vi "Interfaz Control.vi"() -> ()   [LabVIEW 2022 SP3]
uses:
  MQTT/mqtt_lv2013/mqtt Folder/src/class/mqtt/mqttTypedef/mqttSubscribeCluster.ctl
  MQTT/mqtt_lv2013/mqtt Folder/src/class/mqtt/mqttTypedef/mqttQOSlevel.ctl
  MQTT/mqtt_lv2013/mqtt Folder/src/class/mqtt/mqttTypedef/mqttConnectionStatus.ctl
  MQTT/mqtt_lv2013/mqtt Folder/src/class/mqtt/mqttTypedef/mqttConnectionMeta.ctl
  MQTT/mqtt_lv2013/mqtt Folder/src/class/mqtt/mqttTXqueue/mqttTXdataQueueFunction.ctl
  MQTT/mqtt_lv2013/mqtt Folder/src/class/mqtt/mqttConfigFunction.ctl
  MQTT/mqtt_lv2013/mqtt Folder/src/class/mqtt/mqttTXqueue/mqttRXsubscriptionEventFunction.ctl
  MQTT/mqtt_lv2013/mqtt Folder/src/class/mqtt/mqttTypedef/mqttBroker.ctl
  MQTT/mqtt_lv2013/mqtt Folder/src/class/mqtt/mqttTypedef/mqttConnectionFlags.ctl
  MQTT/mqtt_lv2013/mqtt Folder/src/class/mqtt/mqttTypedef/mqttWillInformation.ctl
  MQTT/mqtt_lv2013/mqtt Folder/src/class/mqtt/mqtt.lvclass
panel:
  out "Retirando pieza del escaner":bool
  in  "Numeric 2":u64
  out "Escaner Finalizo":bool
  out "publishMessageID 6":u16 format="%02x"
  in  "connMeta 6":T1
  in  "Home Brazo":bool
  out "String":string
  in  "Ir a":bool
  out "publishMessageID 5":u16 format="%02x"
  in  "connMeta 5":T1
  in  "Horizontal Pointer Slide":u32(slide)
  out "Escaner en proceso":bool
  out "publishMessageID 4":u16 format="%02x"
  in  "connMeta 4":T1
  in  "Selección Pieza a cortar":u16(ring) items=["Ninguna", "1", "2", "3", "4", "5", "6", "7", "8", "9", "10"]
  in  "Selección Pieza a imprimir":u16(ring) items=["Ninguna", "1", "2", "3", "4", "5"]
  in  "Cantidad de piezas a cortar":u16(ring) items=["Ninguna", "1", "2", "3", "4"]
  in  "Cantidad de piezas a imprimir":u16(ring) items=["Ninguna", "1", "2", "3", "4"]
  out "publishMessageID 3":u16 format="%02x"
  in  "connMeta 3":T1
  in  "Pieza a Cortar":u16(ring)
  in  "Pieza a Imprimir":u16(ring)
  in  "quit":bool
  out "Verificar Conexión":bool=TRUE
  in  "pingRequest":bool
  out "messageID":u16
  out "RX Value":string
  out "RX Topic":string
  in  "subscribe":bool
  in  "connect":bool
  out "Colocando pieza en escaner":bool
  out "Retirando pieza del Escaner 3D":bool
  out "Retirando pieza de cortadora Laser":bool
  out "Retirando pieza de Impresora 3D":bool
  out "Brazo en reposo":bool
  out "Br. Soldador en proceso":bool
  out "Pieza Posicionada":bool
  out "Cortadora en proceso":bool
  in  "Detener Impresora 5":bool
  in  "Iniciar Cortadora 6":bool
  in  "Iniciar Cortadora 5":bool
  in  "Iniciar Cortadora 4":bool
  in  "Detener Impresora 4":bool
  in  "Iniciar Escaner":bool
  in  "Detener Impresora 2":bool
  in  "Iniciar Cortadora":bool
  in  "Detener Impresora":bool
  in  "Iniciar Impresora":bool
  out "Impresora Terminó":bool
  out "publishMessageID 2":u16 format="%02x"
  in  "connMeta 2":T1
  out "Activación Proceso":bool
  out "y":string="Test"
  out "Numeric":i32
  in  "disconnect":bool
  out "sessionPresent":bool
  out "connStatus":T3
  in  "subscriptionInfo":T4[](array[typedef])=[{"Topic"="a/b", "QoS"=enum."At most once"}]
  out "subscribeMessageID":u16 format="%02x"
  out "subscribeSuccess":bool
  out "error out":errorcluster
  # "Impresora 3D"
  # "Brazo Manipulador"
  # "Cortadora Láser"
  # "Comunicación con el CIM"
  # "Escaner 3D"
  # "Brazo Soldador"
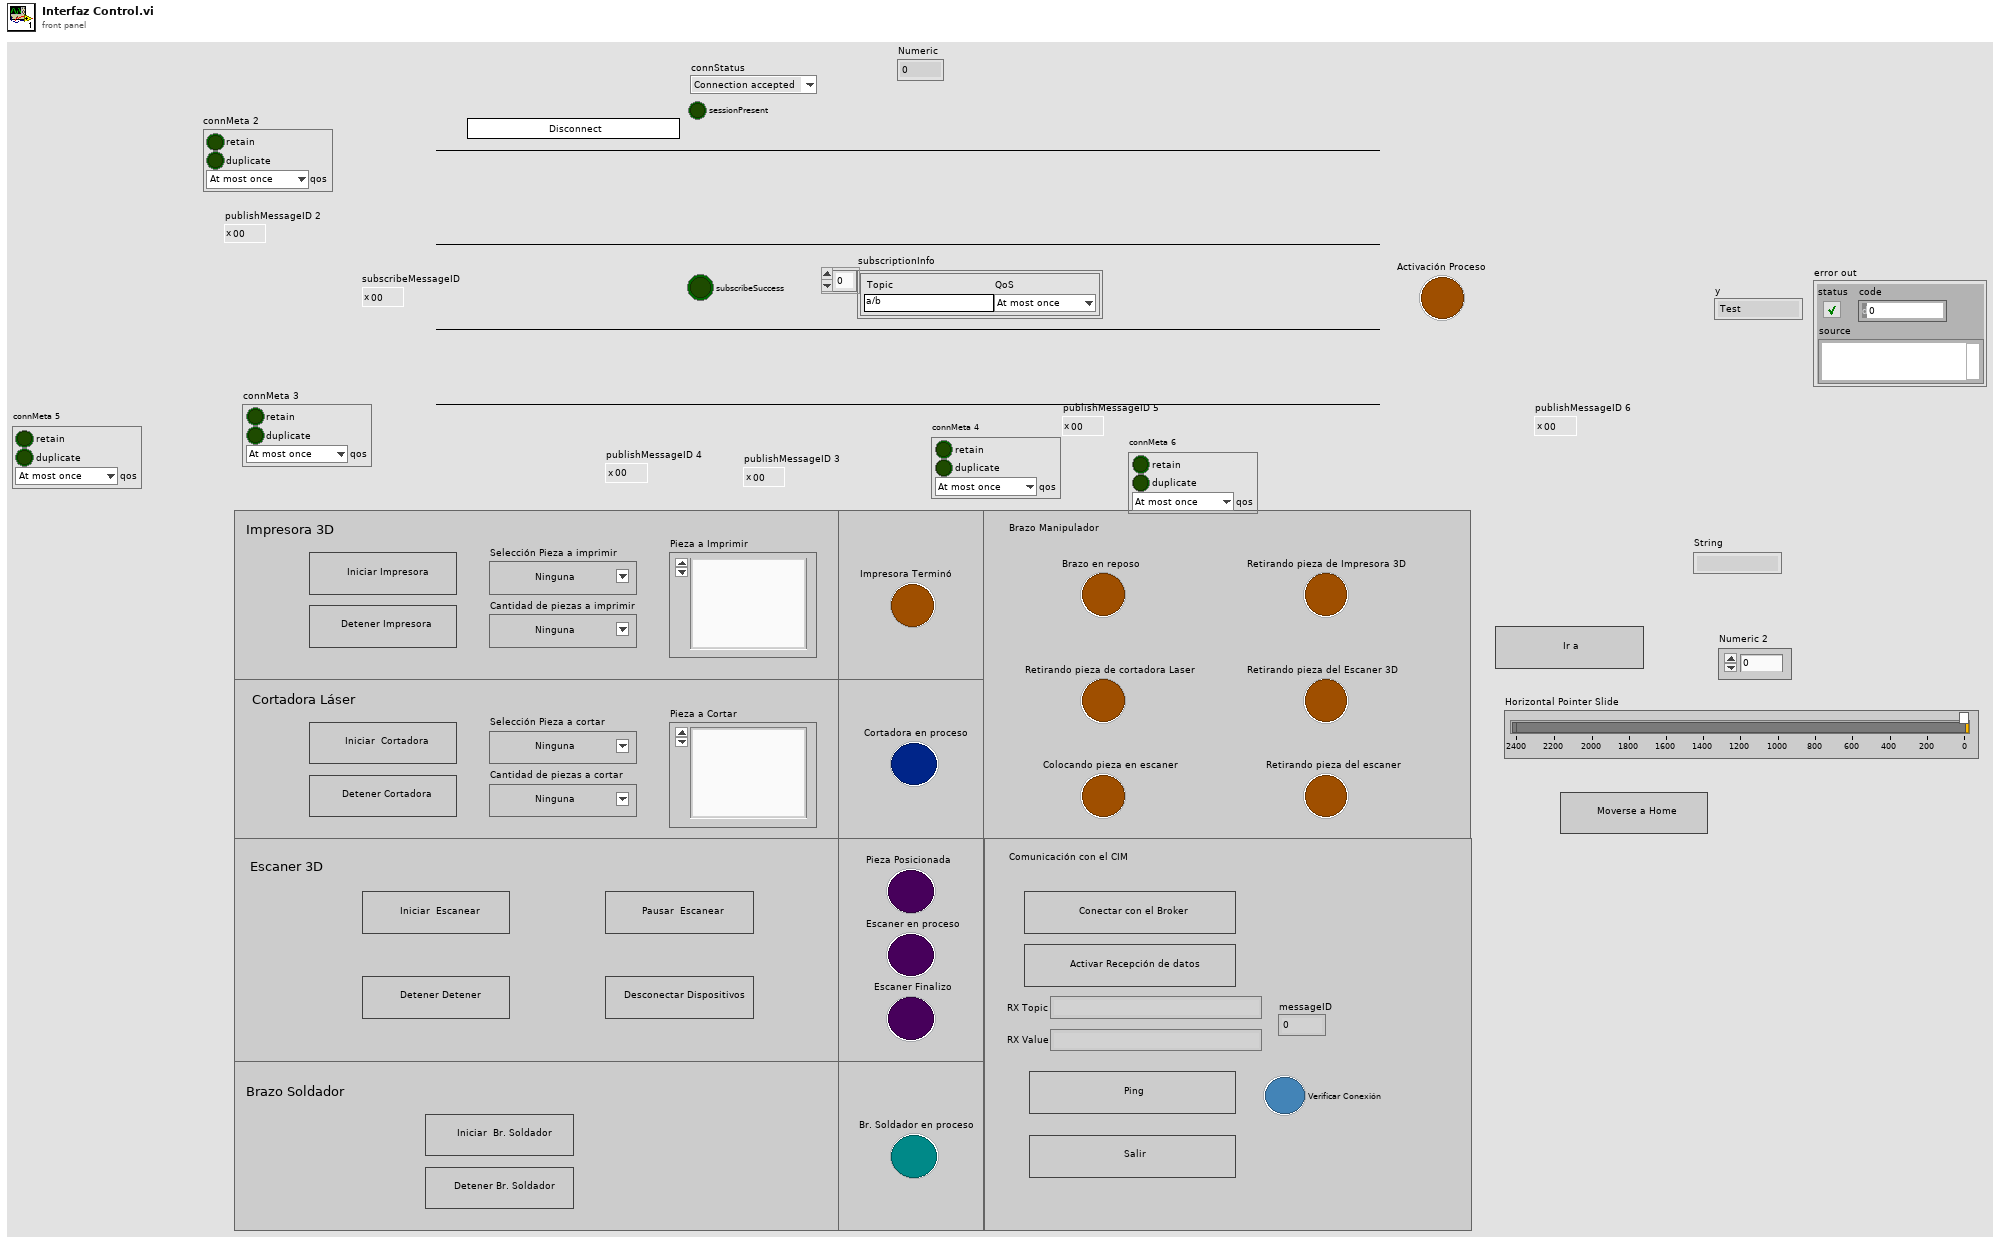
[diagram p1: front panel]
types:
  T1 = typedef "mqttConnectionMeta.ctl" = cluster{"retain":bool, "duplicate":bool, "qos":T2}
  T2 = typedef "mqttQOSlevel.ctl" = enum8{"At most once", "At least once", "Exactly once", "Reserved"}
  T3 = typedef "mqttConnectionStatus.ctl" = enum16{"Connection accepted", "Connection refused: unacceptable protocol version", "Connection refused: identifier rejected", "Connection refused: Server unavailable", "Connection refused: bad user name or password", "Connection refused: not authorized"}
  T4 = typedef "mqttSubscribeCluster.ctl" = cluster{"Topic":string, "QoS":T2}
  T5 = typedef "mqttWillInformation.ctl" = cluster{"User Name":string, "Password":string}
  T6 = typedef "mqttConnectionFlags.ctl" = cluster{"reserved":bool, "clean session":bool, "will flag":bool, "willQOS":enum8{"At most once", "At least once", "Exactly once", "Reserved"}, "will retain":bool, "password":bool, "user name":bool}
  T7 = typedef "mqttBroker.ctl" = cluster{"address":string, "port":u16, "connTimeout":i32, "writeTimeout":i32, "readTimeout":i32, "subTimeout":i32}
  T8 = typedef "mqttRXsubscriptionEventFunction.ctl" = enum16{"init", "deinit", "getEventRef", "event"}
  T9 = typedef "mqtt.lvclass/mqttConfigFunction.ctl" = enum16{"init", "deinit", "set", "get"}
  T10 = typedef "mqttTXdataQueueFunction.ctl" = enum16{"init", "deinit", "getQueue", "enqueue"}
  T11 = enum8{"Enabled", "Disabled", "Disabled and Grayed Out"}
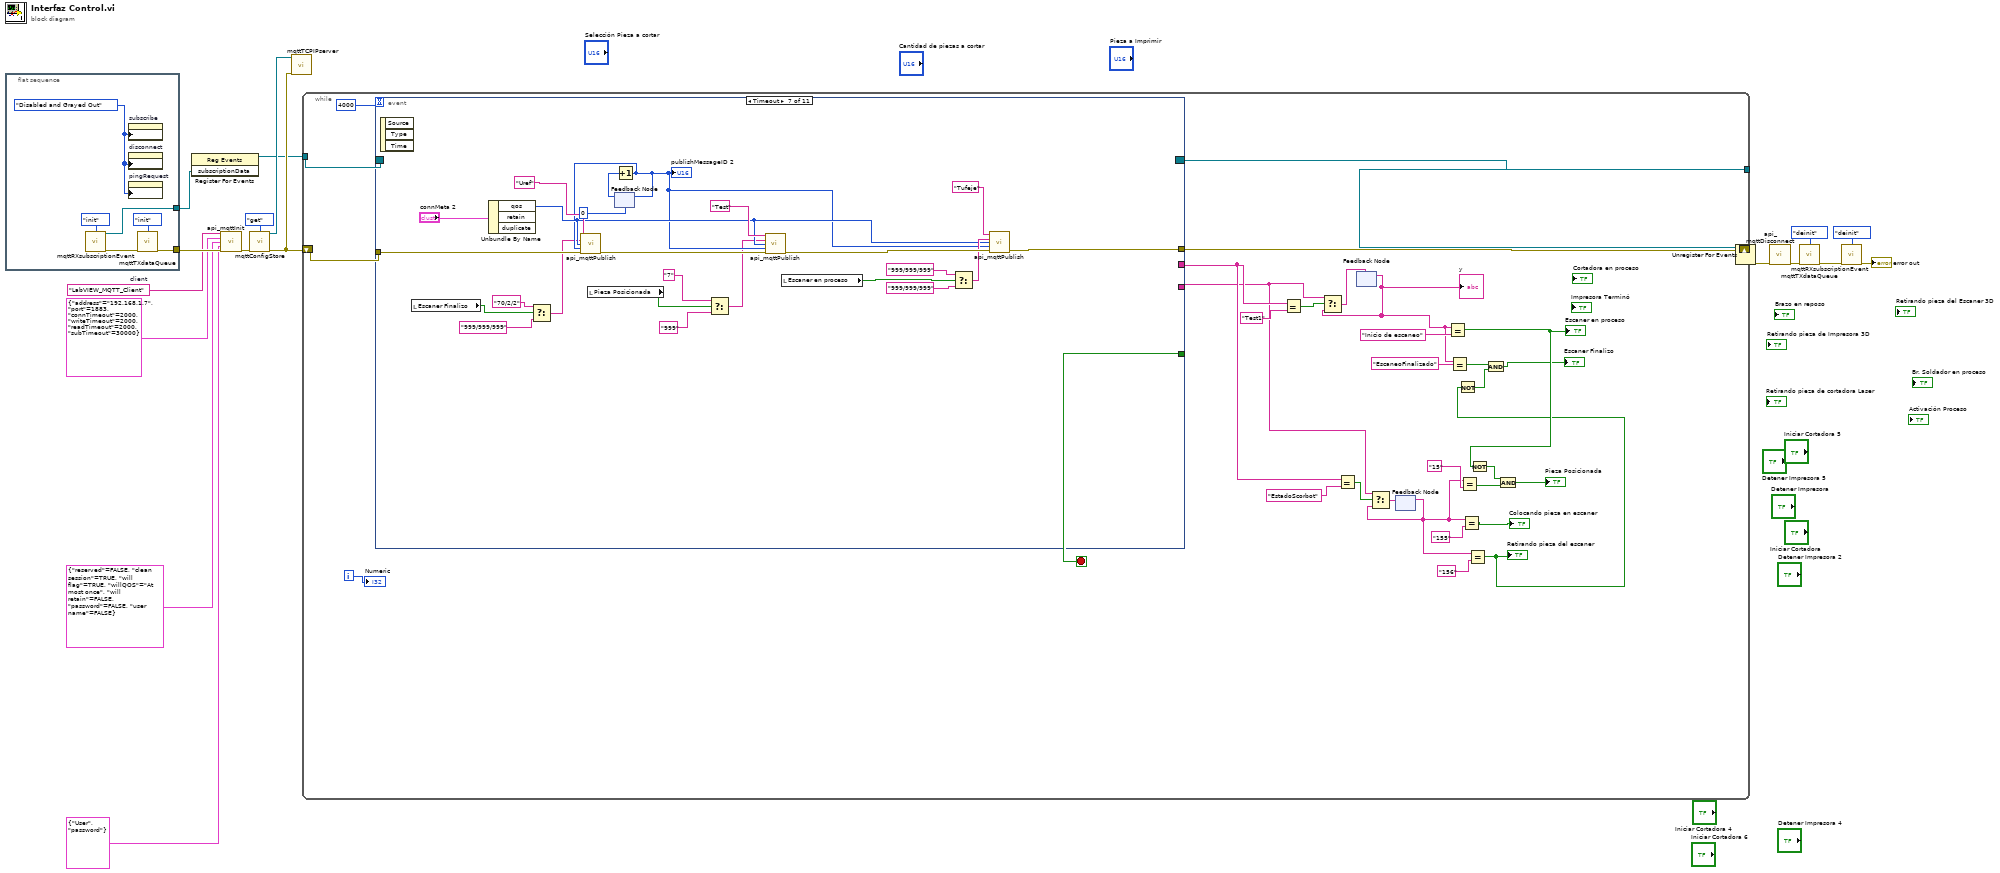
[diagram p0: block diagram]
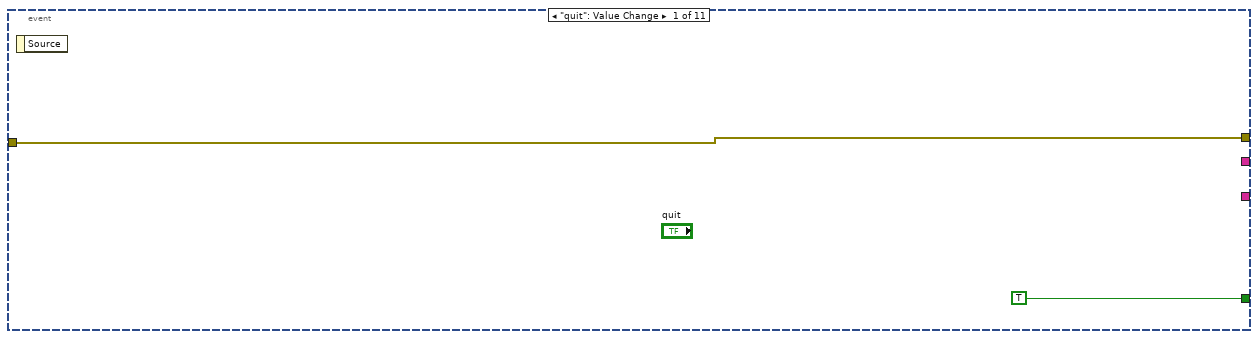
[diagram p2: hidden frame]
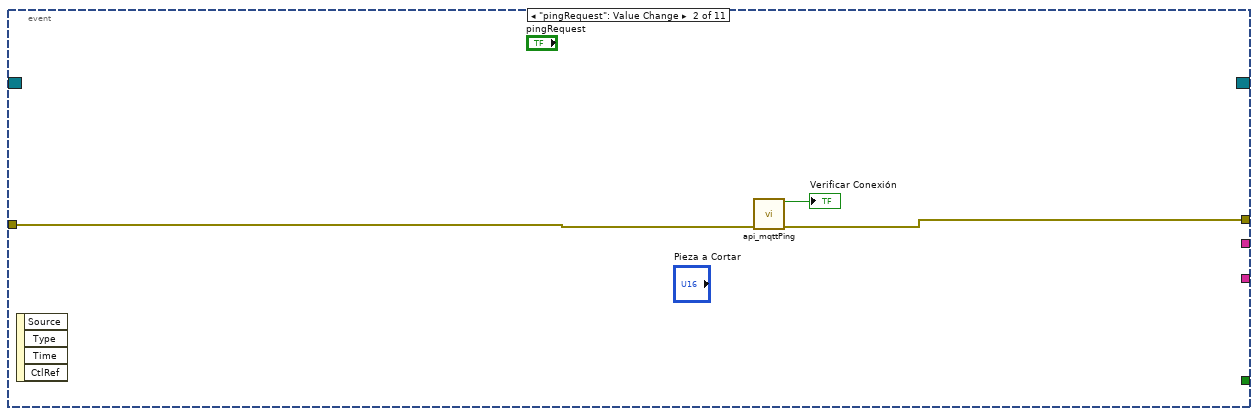
[diagram p3: hidden frame]
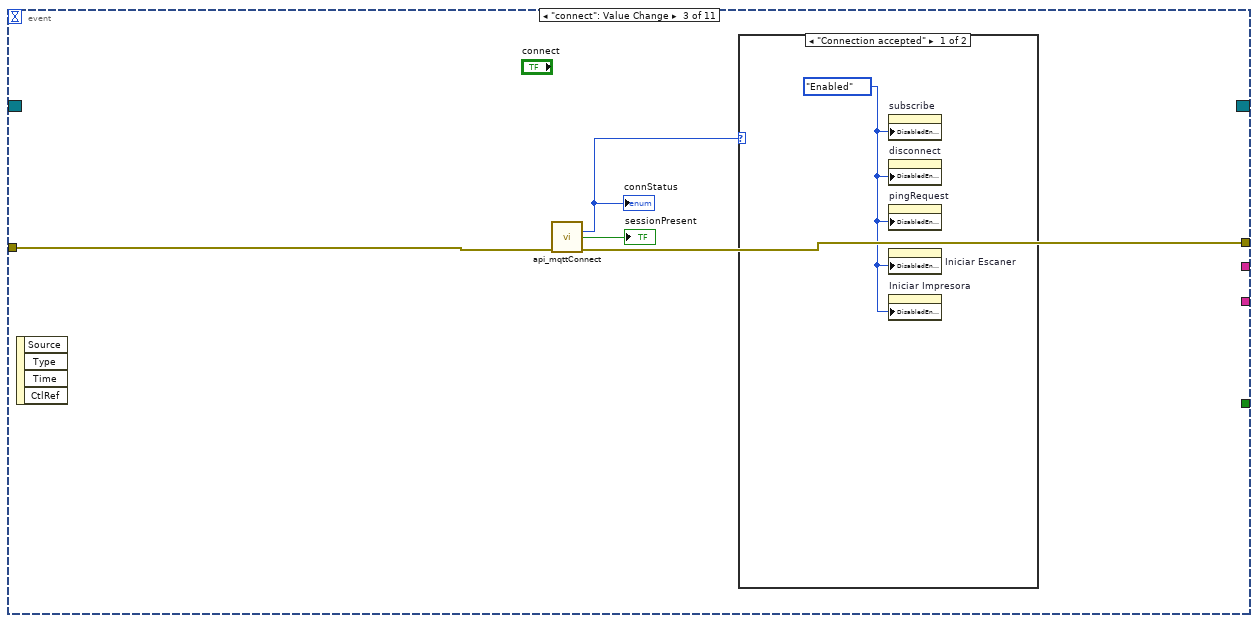
[diagram p4: hidden frame]
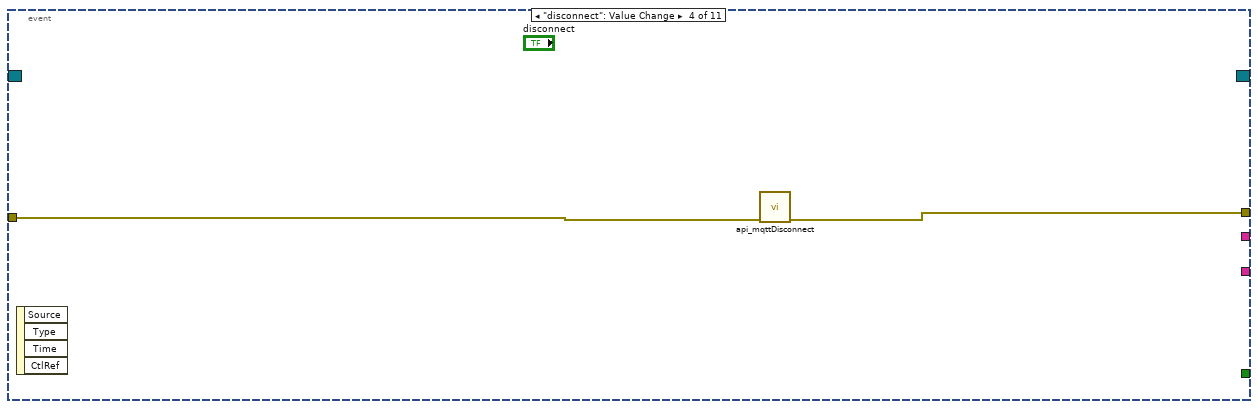
[diagram p6: hidden frame]
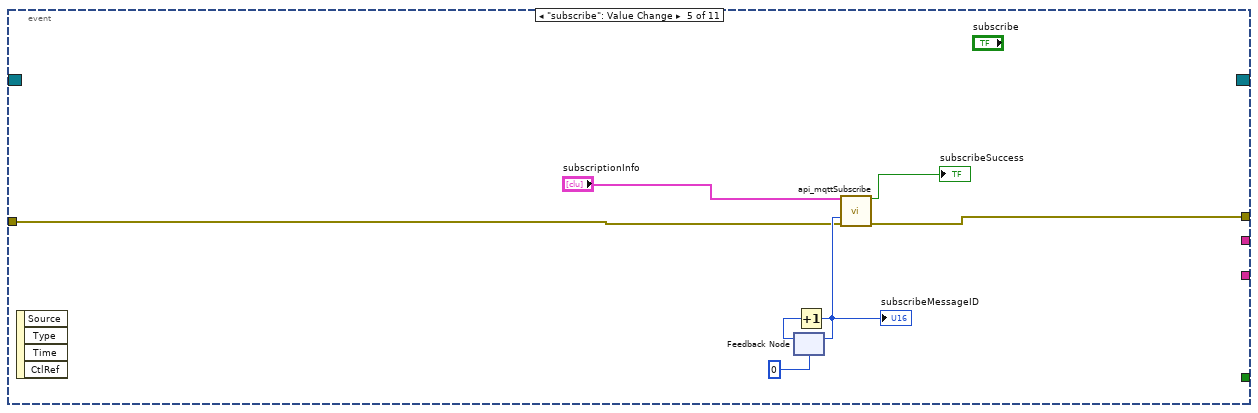
[diagram p7: hidden frame]
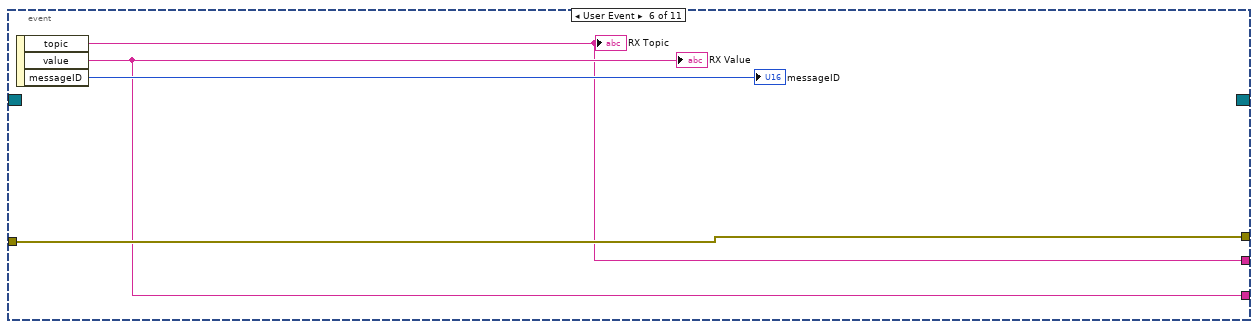
[diagram p8: hidden frame]
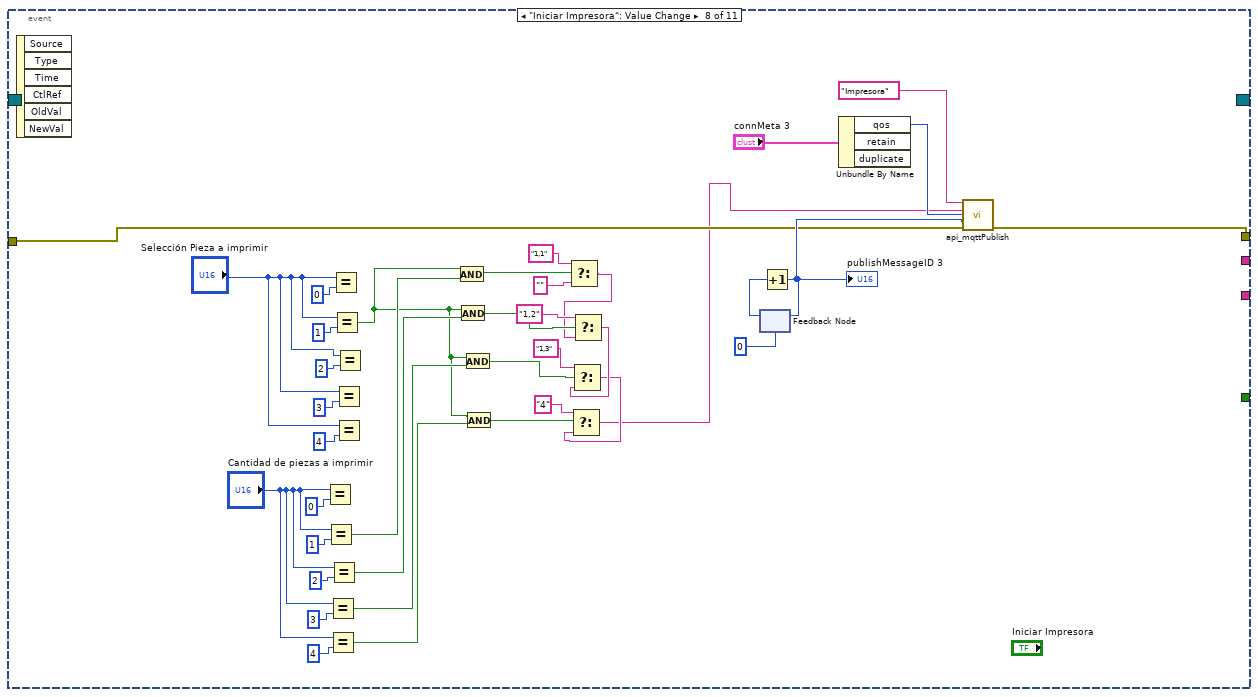
[diagram p9: hidden frame]
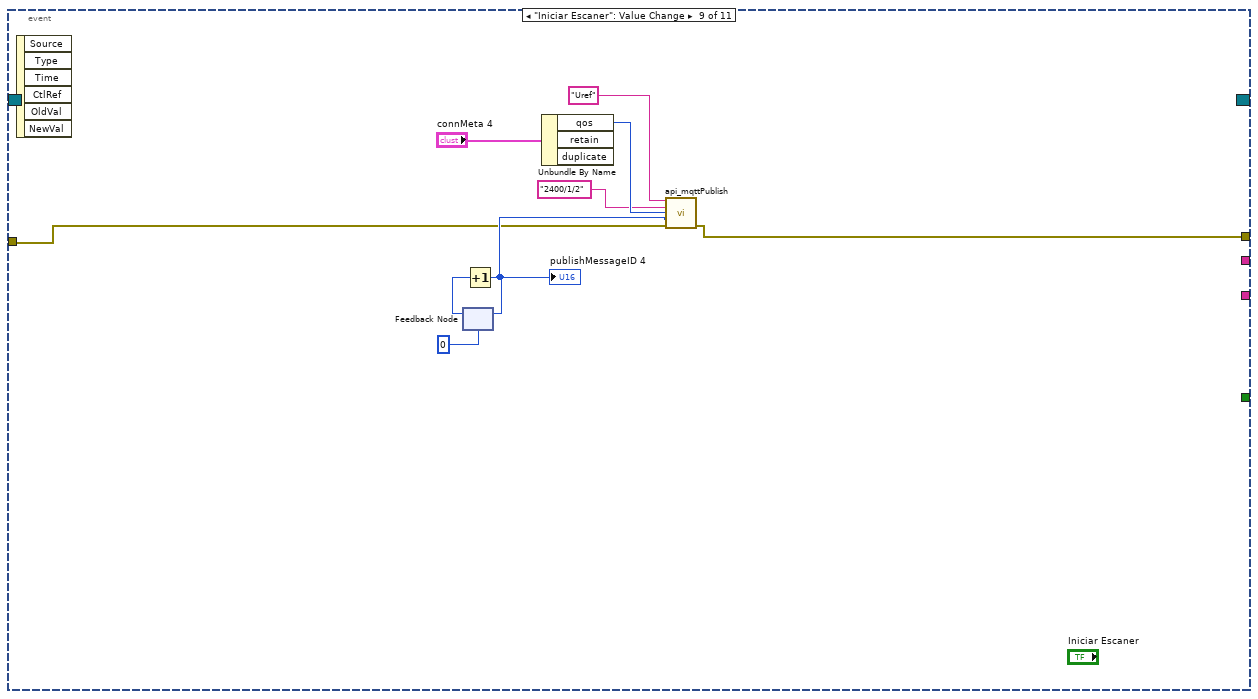
[diagram p10: hidden frame]
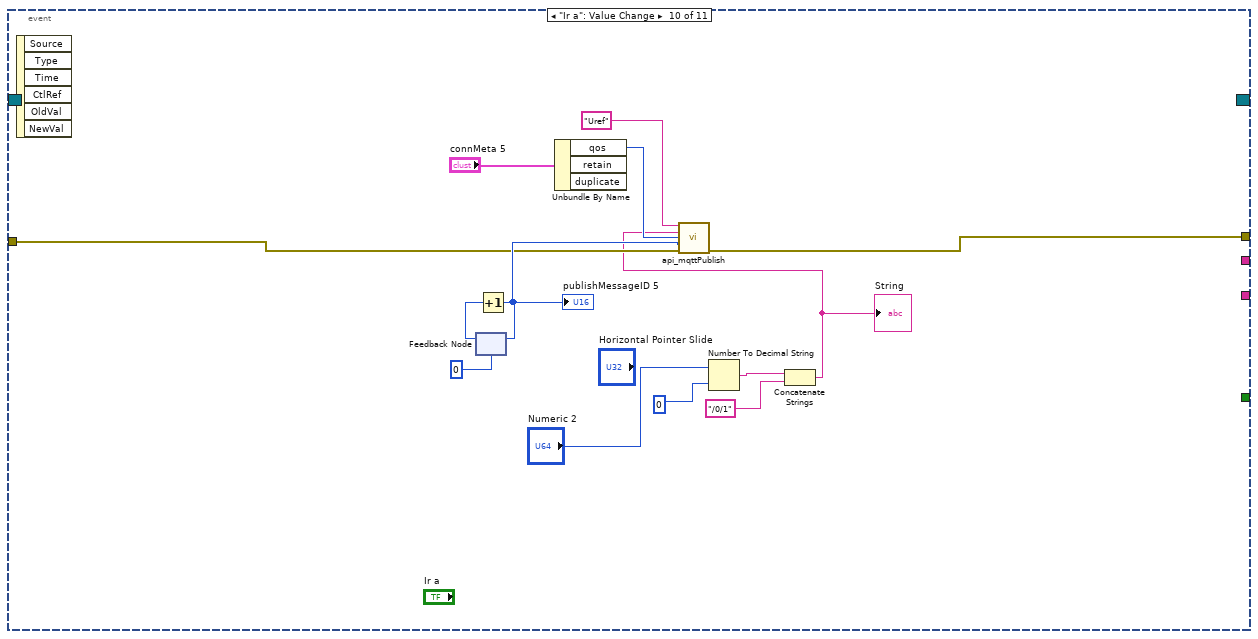
[diagram p11: hidden frame]
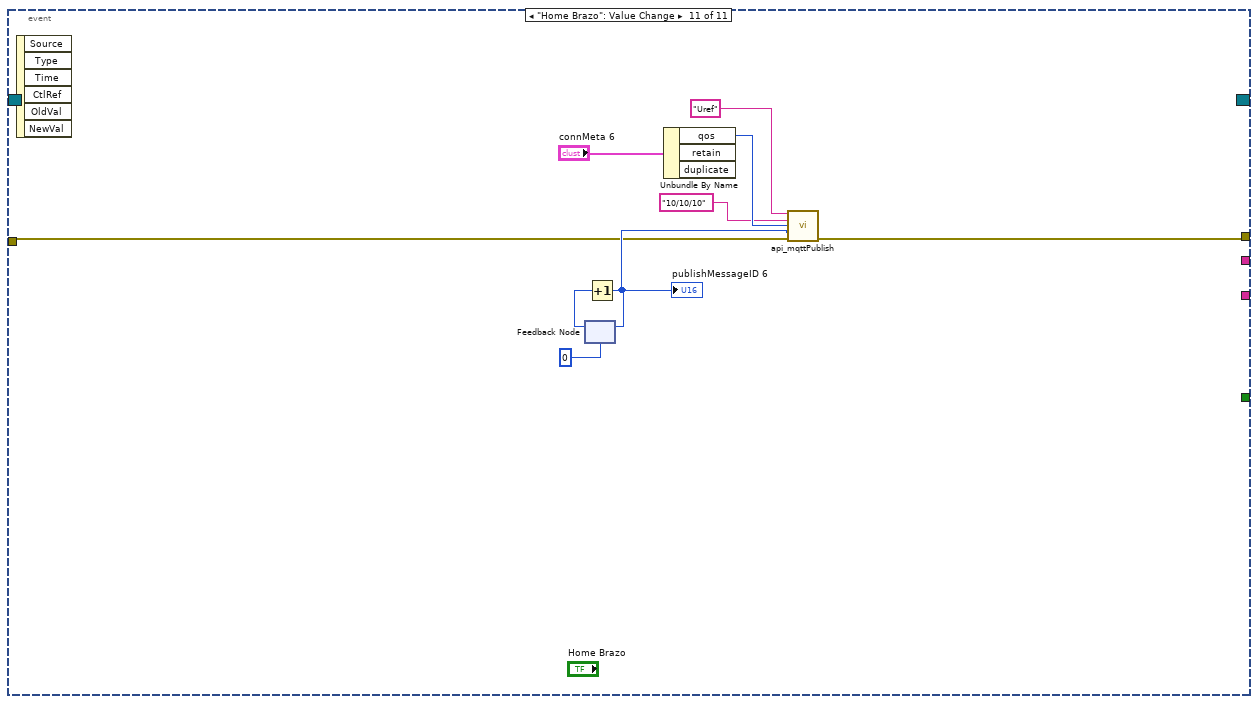
[diagram p12: hidden frame]
diagram:
  w4 = "LabVIEW_MQTT_Client"  # client
  n1 = flat-sequence {
    tunnel: [w24] -> w18
    tunnel: [w21] -> w12
    frame #0 {
      w20 = T11."Disabled and Grayed Out" ("Disabled")
      n2 = call "mqttRXsubscriptionEvent.vi"("function"=mqttRXsubscriptionEventFunction."init") -> ("subscriptionData"=w21:refnum<user-event>, "error out"=w23:errorcluster)  [unwired: 13 in]
      n3 = property on="subscribe" class="Bool"("DisabledEnum"=w20) -> ()  [unwired: 2 in, 2 out]
      n4 = property on="disconnect" class="Bool"("DisabledEnum"=w20) -> ()  [unwired: 2 in, 2 out]
      n5 = property on="pingRequest" class="Bool"("DisabledEnum"=w20) -> ()  [unwired: 2 in, 2 out]
      n6 = call "mqttTXdataQueue.vi"("function"=mqttTXdataQueueFunction."init", "error in (no error)"=w23) -> ("error out"=w24:errorcluster)  [unwired: 12 in, 1 out]
    }
  }
  n7 = register-events(w12) -> (reference out=w11:refnum<event-registration>)  [unwired: 2 in, 1 out]
  n8 = call "api_mqttInit.vi"("client"=w4, "broker"=T7 {"address"="192.168.1.7", "port"=1883, "connTimeout"=2000, "writeTimeout"=2000, "readTimeout"=2000, "subTimeout"=30000}, "connFlags"=T6 {"reserved"=FALSE, "clean session"=TRUE, "will flag"=TRUE, "willQOS"=enum."At most once", "will retain"=FALSE, "password"=FALSE, "user name"=FALSE}, "User Info"=T5 {"User Name"="User", "Password"="password"}, "error in (no error)"=w18) -> ("error out"=w16:errorcluster)  [unwired: 10 in]
  n9 = call "mqttConfigStore.vi"("function"=mqttConfigFunction."get", "error in (no error)"=w16) -> ("mqtt.lvclass out"=w15:refnum<class "mqtt.lvclass">, "error out"=w14:errorcluster)  [unwired: 12 in]
  n10 = call "mqttTCPIPserver.vi"("mqtt.lvclass"=w15, "error in (no error)"=w14) -> ()  [unwired: 12 in, 2 out]
  n11 = while {
    shift-right: [w56] -> w7
    shift-left: w14 -> [w55]
    tunnel: w11 -> [w53]
    tunnel: [w51] -> w5
    i -> [w52]
    stop <- w54 stop-if-true
    n12 = event shown="[6] Timeout" {
      selector: w53 -> [_ _ _ _ _ _ _ _ _ _ _]
      dyn-events: [_ _ _ _ _ _ _ _ _ _ _] -> w51
      timeout: 4000 -> [_ _ _ _ _ _ _ _ _ _ _]
      tunnel: [w57 w60 w64 w67 w71 w79 w85 w135 w143 w156 w165] -> w56
      tunnel: w55 -> [w57 w61 w65 w68 w69 w79 w86 w134 w144 w157 w164]
      tunnel: [TRUE _ _ _ _ _ _ _ _ _ _] -> w54
      tunnel: [_ _ _ _ _ w77 _ _ _ _ _] -> w44
      tunnel: [_ _ _ _ _ w76 _ _ _ _ _] -> w45
      event "quit": Value Change {
        n13 = event-data() -> ()  [unwired: 1 in, 1 out]
      }
      event "pingRequest": Value Change {
        n14 = event-data() -> ()  [unwired: 1 in, 4 out]
        n15 = call "api_mqttPing.vi"("error in (no error)"=w61) -> ("success"=→"Verificar Conexión":bool, "error out"=w60:errorcluster)  [unwired: 13 in]
      }
      event "connect": Value Change {
        n16 = event-data() -> ()  [unwired: 1 in, 4 out]
        n17 = call "api_mqttConnect.vi"("error in (no error)"=w65) -> ("connStatus"=w62:T3, "sessionPresent"=→"sessionPresent":bool, "error out"=w64:errorcluster)  [unwired: 11 in, 1 out]
        "connStatus" <- w62
        n18 = case shown="\"Connection accepted\"" w62 {
          frame "Connection accepted" {
            w66 = T11."Enabled" ("Disabled")
            n19 = property on="subscribe" class="Bool"("DisabledEnum"=w66) -> ()  [unwired: 2 in, 2 out]
            n20 = property on="disconnect" class="Bool"("DisabledEnum"=w66) -> ()  [unwired: 2 in, 2 out]
            n21 = property on="pingRequest" class="Bool"("DisabledEnum"=w66) -> ()  [unwired: 2 in, 2 out]
            n22 = property on="Iniciar Escaner" class="Bool"("DisabledEnum"=w66) -> ()  [unwired: 2 in, 2 out]
            n23 = property on="Iniciar Impresora" class="Bool"("DisabledEnum"=w66) -> ()  [unwired: 2 in, 2 out]
          }
          frame Default {
          }
        }
      }
      event "disconnect": Value Change {
        n24 = event-data() -> ()  [unwired: 1 in, 4 out]
        n25 = call "api_mqttDisconnect.vi"("error in (no error)"=w68) -> ("error out"=w67:errorcluster)  [unwired: 13 in, 1 out]
      }
      event "subscribe": Value Change {
        n26 = event-data() -> ()  [unwired: 1 in, 4 out]
        n27 = feedback #1(u16 0) -> (w74:u16)
        n28 = Increment(x=w74) -> (x+1=w70:u16)
        "subscribeMessageID" <- w70
        n29 = feedback-in #1(w70) -> ()
        n30 = call "api_mqttSubscribe.vi"("subscriptionInfo"="subscriptionInfo", "messageID"=w70, "error in (no error)"=w69) -> ("success"=→"subscribeSuccess":bool, "error out"=w71:errorcluster)  [unwired: 11 in]
      }
      event User Event {
        n31 = event-data() -> ("topic"=w76:string, "value"=w77:string, "messageID"=→"messageID":u16)  [unwired: 1 in]
        "RX Topic" <- w76
        "RX Value" <- w77
      }
      event Timeout {
        n32 = event-data() -> ()  [unwired: 1 in, 3 out]
        n33 = local read "Escaner Finalizo"() -> (w80:bool)
        n34 = Unbundle By Name("connMeta 2") -> ("qos"=w92:T2)  [unwired: 2 out]
        n35 = Select(t="70/2/2", s=w80, f="999/999/999") -> (s? t:f=w81:string)
        n36 = local read "Pieza Posicionada"() -> (w88:bool)
        n37 = feedback #2(u16 0) -> (w101:u16)
        n38 = Increment(x=w101) -> (x+1=w91:u16)
        "publishMessageID 2" <- w91
        n39 = call "api_mqttPublish.vi"("topic"="Uref", "value"=w81, "QoS (At most once)"=w92, "messageID"=w91, "error in (no error)"=w86) -> ("error out"=w87:errorcluster)  [unwired: 9 in, 1 out]
        n40 = feedback-in #2(w91) -> ()
        n41 = Select(t="7", s=w88, f="999") -> (s? t:f=w82:string)
        n42 = call "api_mqttPublish.vi"("topic"="Test", "value"=w82, "QoS (At most once)"=w92, "messageID"=w91, "error in (no error)"=w87) -> ("error out"=w98:errorcluster)  [unwired: 9 in, 1 out]
        n43 = local read "Escaner en proceso"() -> (w89:bool)
        n44 = Select(t="999/999/999", s=w89, f="999/999/999") -> (s? t:f=w94:string)
        n45 = call "api_mqttPublish.vi"("topic"="Tufeje", "value"=w94, "QoS (At most once)"=w92, "messageID"=w91, "error in (no error)"=w98) -> ("error out"=w85:errorcluster)  [unwired: 9 in, 1 out]
      }
      event "Iniciar Impresora": Value Change {
        n46 = event-data() -> ()  [unwired: 1 in, 6 out]
        n47 = Equal?(x="Cantidad de piezas a imprimir", y=u16 0) -> ()  [unwired: 1 out]
        n48 = Equal?(x="Cantidad de piezas a imprimir", y=u16 1) -> (x = y?=w121:bool)
        n49 = Equal?(x="Cantidad de piezas a imprimir", y=u16 3) -> (x = y?=w113:bool)
        n50 = Equal?(x="Cantidad de piezas a imprimir", y=u16 4) -> (x = y?=w108:bool)
        n51 = Equal?(x="Cantidad de piezas a imprimir", y=u16 2) -> (x = y?=w117:bool)
        n52 = Equal?(x="Selección Pieza a imprimir", y=u16 0) -> ()  [unwired: 1 out]
        n53 = Equal?(x="Selección Pieza a imprimir", y=u16 1) -> (x = y?=w109:bool)
        n54 = Equal?(x="Selección Pieza a imprimir", y=u16 3) -> ()  [unwired: 1 out]
        n55 = Equal?(x="Selección Pieza a imprimir", y=u16 4) -> ()  [unwired: 1 out]
        n56 = Equal?(x="Selección Pieza a imprimir", y=u16 2) -> ()  [unwired: 1 out]
        n57 = And(x=w109, y=w121) -> (x .and. y?=w120:bool)
        n58 = And(x=w109, y=w117) -> (x .and. y?=w115:bool)
        n59 = And(x=w109, y=w113) -> (x .and. y?=w110:bool)
        n60 = And(x=w109, y=w108) -> (x .and. y?=w107:bool)
        n61 = Select(t="1,1", s=w120, f="") -> (s? t:f=w114:string)
        n62 = Select(t="1,2", s=w115, f=w114) -> (s? t:f=w111:string)
        n63 = Select(t="1,3", s=w110, f=w111) -> (s? t:f=w106:string)
        n64 = Select(t="4", s=w107, f=w106) -> (s? t:f=w104:string)
        n65 = feedback #3(u16 0) -> (w138:u16)
        n66 = Increment(x=w138) -> (x+1=w137:u16)
        "publishMessageID 3" <- w137
        n67 = feedback-in #3(w137) -> ()
        n68 = Unbundle By Name("connMeta 3") -> ("qos"=w140:T2)  [unwired: 2 out]
        n69 = call "api_mqttPublish.vi"("topic"="Impresora", "value"=w104, "QoS (At most once)"=w140, "messageID"=w137, "error in (no error)"=w134) -> ("error out"=w135:errorcluster)  [unwired: 9 in, 1 out]
      }
      event "Iniciar Escaner": Value Change {
        n70 = event-data() -> ()  [unwired: 1 in, 6 out]
        n71 = feedback #4(u16 0) -> (w147:u16)
        n72 = Increment(x=w147) -> (x+1=w146:u16)
        "publishMessageID 4" <- w146
        n73 = feedback-in #4(w146) -> ()
        n74 = Unbundle By Name("connMeta 4") -> ("qos"=w149:T2)  [unwired: 2 out]
        n75 = call "api_mqttPublish.vi"("topic"="Uref", "value"="2400/1/2", "QoS (At most once)"=w149, "messageID"=w146, "error in (no error)"=w144) -> ("error out"=w143:errorcluster)  [unwired: 9 in, 1 out]
      }
      event "Ir a": Value Change {
        n76 = event-data() -> ()  [unwired: 1 in, 6 out]
        n77 = feedback #5(u16 0) -> (w160:u16)
        n78 = Increment(x=w160) -> (x+1=w159:u16)
        "publishMessageID 5" <- w159
        n79 = feedback-in #5(w159) -> ()
        n80 = Unbundle By Name("connMeta 5") -> ("qos"=w162:T2)  [unwired: 2 out]
        n81 = Number To Decimal String(number="Numeric 2", width (-)=i16 0) -> (decimal integer string=w154:string)
        n82 = Concatenate Strings(w154, "/0/1" ("string")) -> (w152:string)
        "String" <- w152
        n83 = call "api_mqttPublish.vi"("topic"="Uref", "value"=w152, "QoS (At most once)"=w162, "messageID"=w159, "error in (no error)"=w157) -> ("error out"=w156:errorcluster)  [unwired: 9 in, 1 out]
      }
      event "Home Brazo": Value Change {
        n84 = event-data() -> ()  [unwired: 1 in, 6 out]
        n85 = feedback #6(u16 0) -> (w169:u16)
        n86 = Increment(x=w169) -> (x+1=w168:u16)
        "publishMessageID 6" <- w168
        n87 = feedback-in #6(w168) -> ()
        n88 = Unbundle By Name("connMeta 6") -> ("qos"=w171:T2)  [unwired: 2 out]
        n89 = call "api_mqttPublish.vi"("topic"="Uref", "value"="10/10/10", "QoS (At most once)"=w171, "messageID"=w168, "error in (no error)"=w164) -> ("error out"=w165:errorcluster)  [unwired: 9 in, 1 out]
      }
    }
    n90 = Equal?(x=w45, y="Test1") -> (x = y?=w50:bool)
    n91 = Equal?(x=w45, y="EstadoScorbot") -> (x = y?=w43:bool)
    n92 = feedback #7() -> (w34:string)  [unwired: 1 in]
    "y" <- w34
    n93 = Select(t=w44, s=w50, f=w34) -> (s? t:f=w48:string)
    n94 = feedback-in #7(w48) -> ()
    n95 = feedback #8() -> (w30:string)  [unwired: 1 in]
    n96 = Select(t=w44, s=w43, f=w30) -> (s? t:f=w39:string)
    n97 = feedback-in #8(w39) -> ()
    n98 = Equal?(x=w34, y="Inicio de escaneo") -> (x = y?=w35:bool)
    "Escaner en proceso" <- w35
    n99 = Equal?(x=w34, y="EscaneoFinalizado") -> (x = y?=w29:bool)
    n100 = Equal?(x=w30, y="15") -> (x = y?=w37:bool)
    n101 = Equal?(x=w30, y="155") -> (x = y?=→"Colocando pieza en escaner":bool)
    n102 = Equal?(x=w30, y="156") -> (x = y?=w26:bool)
    "Retirando pieza del escaner" <- w26
    n103 = Not(x=w26) -> (.not. x?=w27:bool)
    n104 = Not(x=w35) -> (.not. x?=w36:bool)
    n105 = And(x=w29, y=w27) -> (x .and. y?=→"Escaner Finalizo":bool)
    n106 = And(x=w36, y=w37) -> (x .and. y?=→"Pieza Posicionada":bool)
    "Numeric" <- w52
  }
  n107 = Unregister For Events(event registration refnum=w5, error in=w7) -> (error out=w6:errorcluster)
  n108 = call "api_mqttDisconnect.vi"("error in (no error)"=w6) -> ("error out"=w13:errorcluster)  [unwired: 13 in, 1 out]
  n109 = call "mqttTXdataQueue.vi"("function"=mqttTXdataQueueFunction."deinit", "error in (no error)"=w13) -> ("error out"=w9:errorcluster)  [unwired: 12 in, 1 out]
  n110 = call "mqttRXsubscriptionEvent.vi"("function"=mqttRXsubscriptionEventFunction."deinit", "error in (no error)"=w9) -> ("error out"=→"error out":errorcluster)  [unwired: 12 in, 1 out]
